vi "Constants.vi"() -> ()   [LabVIEW 2017, in "Switch Shared.lvlib"]
doc: "Use this Global VI to access the GUIDs assigned to the page resources of the Custom Device."
uses:
  Switch Shared.lvlib
panel:
  in  "Tab Control":enum32{"GUIDS", "Constants", "Properties"}(tab)
  in  "RAFCD_Switch":string="afbe9d59-42ef-4901-90cd-ae7efbb062d7"
  in  "Compiled.Settings":string="Compiled.Settings"
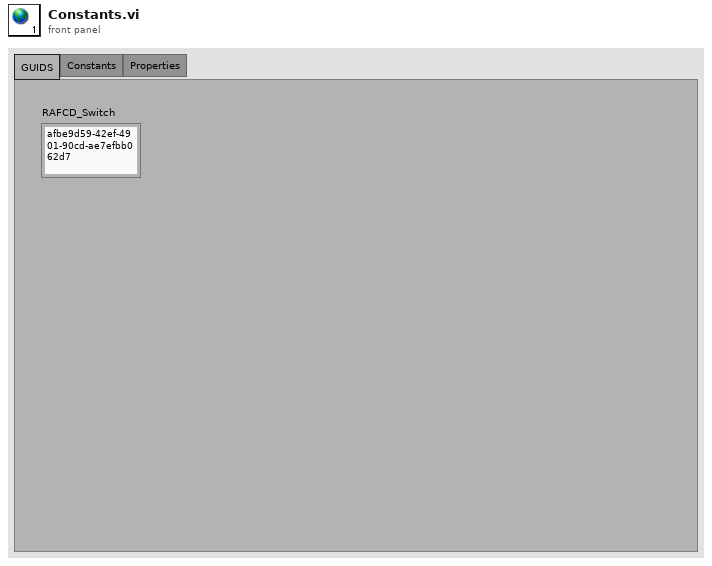
[diagram p1: front panel]
diagram:
